vi "Romi-Drive-System-Get-Max-Speed.vi"() -> (3 "MaxSpeed-Ft/Sec":dbl)   [LabVIEW 2019]
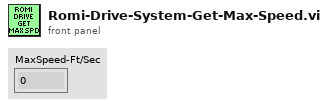
[diagram p1: front panel]
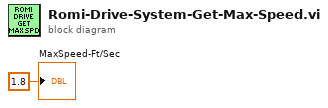
[diagram p0: block diagram]
diagram:
  "MaxSpeed-Ft/Sec" <- 1.8 ("MaxSpeed-Ft/Sec")
